vi "Reorder Schedule(Prins FIFO) based on Start Times.vi"(11 "Start Times (MxJ)":i32[][](array[numeric])) -> (3 "Reordered Schedule(Prins FIFO)":u16[](array[numeric]))   [LabVIEW 2013]
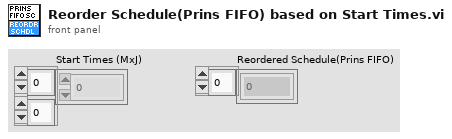
[diagram p1: front panel]
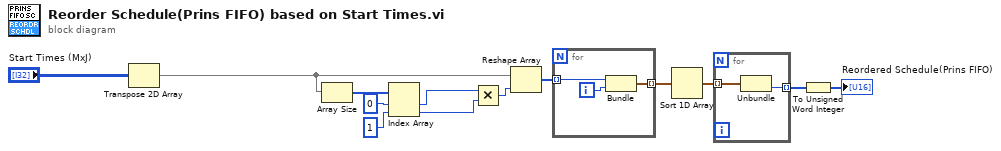
[diagram p0: block diagram]
diagram:
  n1 = Transpose 2D Array(2D array="Start Times (MxJ)") -> (transposed array=w7:i32[][])
  n2 = Array Size(array=w7) -> (size(s)=w12:i32[])
  n3 = Index Array(array=w12, index #1=0 ("index"), index #2=1 ("index")) -> (element #1=w9:i32, element #2=w8:i32)
  n4 = Multiply(x=w9, y=w8) -> (x*y=w6:i32)
  n5 = Reshape Array(w7, w6) -> (w5:i32[])
  n6 = for {
    tunnel: w5 -> [w16] mode=indexing
    tunnel: [w14] -> w4 mode=indexing
    i -> [w15]
    n7 = Bundle(w16, w15) -> (w14:cluster{i32, i32})  [unwired: 1 in]
  }
  n8 = Sort 1D Array(array=w4) -> (sorted array=w3:cluster{i32, i32}[])
  n9 = for {
    tunnel: w3 -> [w18] mode=indexing
    tunnel: [w17] -> w2 mode=indexing
    n10 = Unbundle(w18) -> (w17:i32)  [unwired: 1 out]
  }
  n11 = To Unsigned Word Integer(number=w2) -> (unsigned 16bit integer=→"Reordered Schedule(Prins FIFO)":u16[])
